vi "Device ID to Name.vi"(8 "Error In":errorcluster, 9 "Device ID":u8, 10 "Device Family":T4, 11 "LINX Device Config":T5) -> (0 "Error Out":errorcluster, 2 "Device Name":string, 3 "LINX Device Config":T5)   [LabVIEW 2011, in "LVH-LINX.lvlib" / "Device.lvlib"]
doc: "Get the device name from the device family and device ID. Store in LINX Device Config cluster and return device name."
uses:
  Device.lvlib
  Type Defs/LINX Device Config.ctl
  Type Defs/Interface.ctl
  Type Defs/TCP Config.ctl
  Type Defs/Device Family.ctl
  Type Defs/Devices - Digilent.ctl
  Type Defs/Devices - NI.ctl
  Type Defs/Devices - Arduino.ctl
  LVH-LINX.lvlib
panel:
  in  "Arduino Device":T1
  in  "NI Device":T2
  in  "Digilent Device":T3
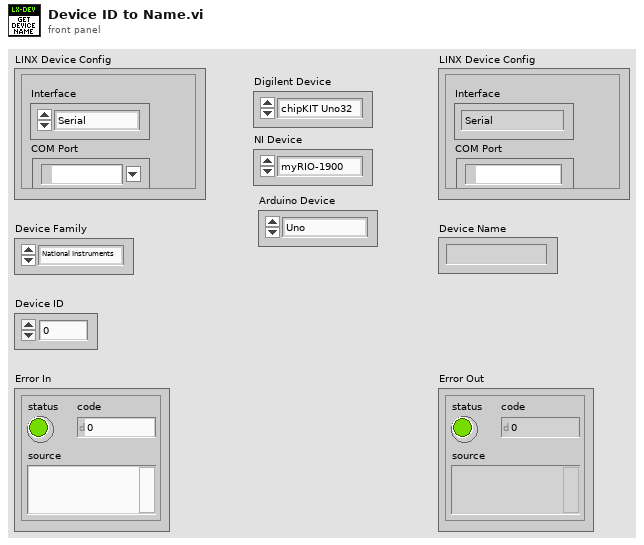
[diagram p1: front panel]
types:
  T1 = typedef "LVH-LINX.lvlib/Devices - Arduino.ctl" = enum16{"Uno", "Mega 2560", "Leonardo", "Due", "Yun", "Nano", "Pro Mini", "Pro", "Fio"}
  T2 = typedef "LVH-LINX.lvlib/Devices - NI.ctl" = enum16{"myRIO-1900", "myRIO-1950"}
  T3 = typedef "LVH-LINX.lvlib/Devices - Digilent.ctl" = enum16{"chipKIT Uno32", "chipKIT uC32", "chipKIT Max32", "chipKIT DP32"}
  T4 = typedef "LVH-LINX.lvlib/Device Family.ctl" = enum8{"National Instruments", "Digilent", "Arduino"}
  T5 = typedef "LVH-LINX.lvlib/Device.lvlib/LINX Device Config.ctl" = cluster{"Interface":T6, "COM Port":refnum<visa-resource-name>, "TCP Configuration":T7, "Device ID":u8, "Device Name":string, "Device Family":T4}
  T6 = typedef "LVH-LINX.lvlib/Interface.ctl" = enum16{"Serial", "TCP"}
  T7 = typedef "LVH-LINX.lvlib/Device.lvlib/TCP Config.ctl" = cluster{"IP Address":string, "Port":dbl}
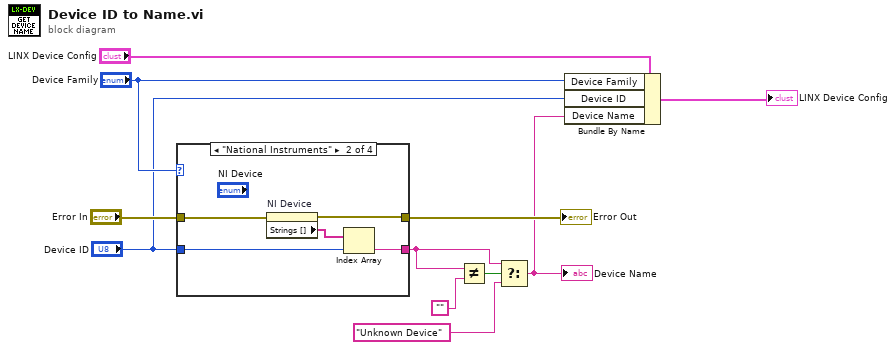
[diagram p0: block diagram]
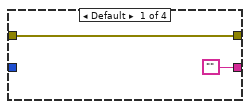
[diagram p2: hidden frame]
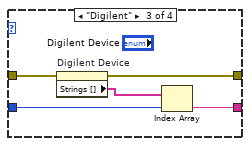
[diagram p3: hidden frame]
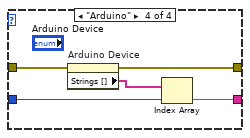
[diagram p4: hidden frame]
diagram:
  n1 = case shown="\"National Instruments\"" "Device Family" {
    tunnel: "Error In" -> [w13 w17 w23 w26]
    tunnel: "Device ID" -> [_ w14 w21 w28]
    tunnel: ["" w15 w20 w27] -> w5
    tunnel: [w13 w18 w19 w25] -> w3
    frame Default {
    }
    frame "National Instruments" {
      n2 = property on="NI Device" class="Enum (strict)"(error in=w17) -> (error out=w18:errorcluster, "Strings []"=w16:string[])  [unwired: 1 in, 1 out]
      n3 = Index Array(array=w16, index=w14) -> (element=w15:string)
    }
    frame "Digilent" {
      n4 = property on="Digilent Device" class="Enum (strict)"(error in=w23) -> (error out=w19:errorcluster, "Strings []"=w22:string[])  [unwired: 1 in, 1 out]
      n5 = Index Array(array=w22, index=w21) -> (element=w20:string)
    }
    frame "Arduino" {
      n6 = property on="Arduino Device" class="Enum (strict)"(error in=w26) -> (error out=w25:errorcluster, "Strings []"=w24:string[])  [unwired: 1 in, 1 out]
      n7 = Index Array(array=w24, index=w28) -> (element=w27:string)
    }
  }
  "Error Out" <- w3
  n8 = Not Equal?(x=w5, y="") -> (x != y?=w6:bool)
  n9 = Select(t=w5, s=w6, f="Unknown Device") -> (s? t:f=w1:string)
  "Device Name" <- w1
  n10 = Bundle By Name(cluster="LINX Device Config", "Device Family"="Device Family", "Device ID"="Device ID", "Device Name"=w1) -> (→"LINX Device Config":T5)
